vi "PhDemoLV.vi"() -> ()   [LabVIEW 2013]
doc: "This is an example VI that demonstrates a few capabilities of the Vision Research Phantom Series LabVIEW Driver."
uses:
  _Type Defs/enum buttons.ctl
  _Type Defs/Point.ctl
  _Type Defs/StampTime.ctl
  _Type Defs/Cine Source.ctl
  _Type Defs/PHCon ACQUIPARAMS.ctl
  _Type Defs/PhCon SyncImaging.ctl
  _Type Defs/Rect.ctl
  _Type Defs/PHCon Time64.ctl
  _Type Defs/PhInt CFA.ctl
  _Type Defs/PhCon Predefined Cines.ctl
  _Type Defs/PhFile InfName.ctl
  _Type Defs/PHCon IMRANGE.ctl
  _Type Defs/PhInt PhProcessImage Selectors.ctl
  Instance          21 27Saved   Application Example .vi
  VRI.lvlib
panel:
  out "Parameters":T1 {"CFA"."CFA" items=["CFA_NONE", "CFA_VRI", "CFA_VRIV6", "CFA_BAYER", "CFA_BAYERFLIP"]; "TriggerTime"."fractions" format="%32.0f"}
  in  "Cine Number":i32=1 max=1
  out "Current Image #":i32
  out "Slide":dbl(slide) scale=0.0..1.0
  in  "Play/Pause":bool
  in  "Preview Img":bool
  in  "Delay (ms)":u32=10
  out "Image Count":u32
  out "Post-Trigger Frames":i32
  in  "Source":T6 items=["Camera RAM", "File"]
  in  "Save Cine":bool
  in  "Open Cine":bool
  in  "Trigger":bool
  in  "Capture":bool
  in  "EXIT":bool
  out "pCameraName":string
  out "pSerial":u32
  in  "Update":bool
  in  "ACQUIPARAMS Display":T7
  in  "Save StampTime":T8
  out "Preview":picture
  out "Continue":bool
  out "Save Progress":u8(slide) max=100 scale=0.0..100.0
  out "active":string="Not Running..."
  out "CAR":T9[](array[typedef])
  in  "Camera Number":u32
  out "error out":errorcluster
  in  "error in":errorcluster
  in  "Current State":T10
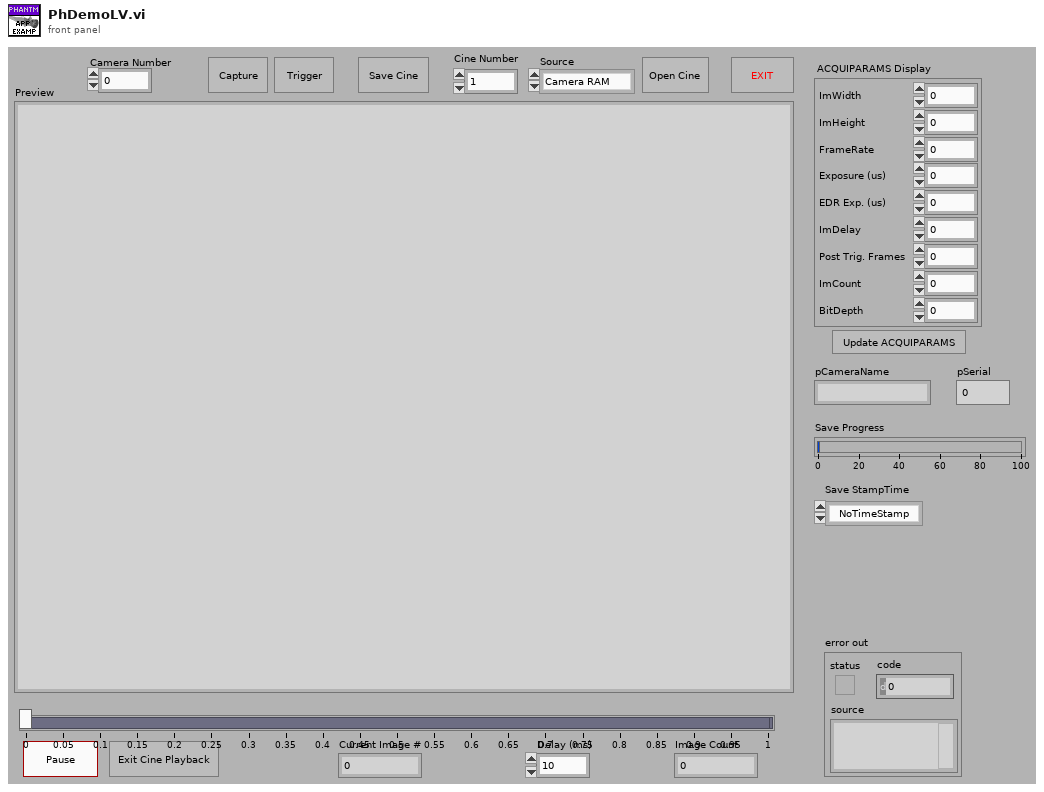
[diagram p1: front panel]
types:
  T1 = typedef "VRI.lvlib/PHCon ACQUIPARAMS.ctl" = cluster{"ImWidth":u32, "ImHeight":u32, "(deprecated)FrameRateInt":u32, "Exposure":u32, "EDRExposure":u32, "ImDelay":u32, "PTFrames":u32, "ImCount":u32, "SyncImaging":T2, "AutoExposure":u32, "AutoExpLevel":u32, "AutoExpSpeed":u32, "AutoExpRect":T3, "Recorded":bool, "TriggerTime":T4, "RecordedCount":u32, "FirstIm":i32, "FRPSteps":u32, "FRPImgNr":i32[], "FRPRate":u32[], "FRPExp":u32[], "Decimation":u32, "BitDepth":u32, "CamGainRed":u32, "CamGainGreen":u32, "CamGainBlue":u32, "CamGain":u32, "ShutterOff":bool, "CFA":T5, "CineName[256]":u8[], "Description[4096]":u8[], "FRPShape [16]":u32[], "dFrameRate":dbl}
  T2 = typedef "VRI.lvlib/PhCon SyncImaging.ctl" = enum32{"SYNC_INTERNAL", "SYNC_EXTERNAL", "SYNC_LOCKTOIRIG"}
  T3 = typedef "VRI.lvlib/Rect.ctl" = cluster{"X":i32, "Y":i32, "Width":i32, "Height":i32}
  T4 = typedef "VRI.lvlib/PHCon Time64.ctl" = cluster{"fractions":u32, "seconds":u32}
  T5 = typedef "VRI.lvlib/PhInt CFA.ctl" = cluster{"CFA":u32, "VRIV6 Mask":cluster{"TL_GRAY":bool, "TR_GRAY":bool, "BL_GRAY":bool, "BR_GRAY":bool}}
  T6 = typedef "VRI.lvlib/Cine Source.ctl" = u16
  T7 = cluster{"ImWidth":u32, "ImHeight":u32, "FrameRate":u32, "Exposure (us)":u32, "EDR Exp. (us)":u32, "ImDelay":u32, "Post Trig. Frames":u32, "ImCount":u32, "BitDepth":u32}
  T8 = typedef "VRI.lvlib/StampTime.ctl" = enum32{"NoTimeStamp", "Time stamp", "", "Time stamp from trigger"}
  T9 = typedef "VRI.lvlib/Point.ctl" = cluster{"X":i32, "Y":i32}
  T10 = typedef "VRI.lvlib/enum buttons.ctl" = enum16{"Initialize", "Wait for Action", "Update", "Capture", "Trigger", "Open Cine", "Save Cine", "End"}
  T11 = typedef "VRI.lvlib/PHCon IMRANGE.ctl" = cluster{"First":i32, "Cnt":u32}
  T12 = typedef "VRI.lvlib/PhCon Predefined Cines.ctl" = i32
  T13 = typedef "VRI.lvlib/PhInt PhProcessImage Selectors.ctl" = u16
  T14 = typedef "VRI.lvlib/PhFile InfName.ctl" = u32
  T15 = typedef "VRI.lvlib/PhInt IH.ctl" = cluster{"biSize":u32, "biWidth":i32, "biHeight":i32, "biPlanes":u16, "biBitCount":u16, "biCompresssion":u32, "biSizeImage":u32, "biXPelsPerMeter":i32, "biYPelsPerMeter":i32, "biClrUsed":u32, "biClrImportant":u32, "BlackLevel":i32, "WhiteLevel":i32}
  T16 = typedef "VRI.lvlib/BITMAPINFOHEADER.ctl" = cluster{"biSize":u32, "biWidth":i32, "biHeight":i32, "biPlanes":u16, "biBitCount":u16, "biCompression":u32, "biSizeImage":u32, "biXPelsPerMeter":i32, "biYPelsPerMeter":i32, "biClrUsed":u32, "biClrImportant":u32}
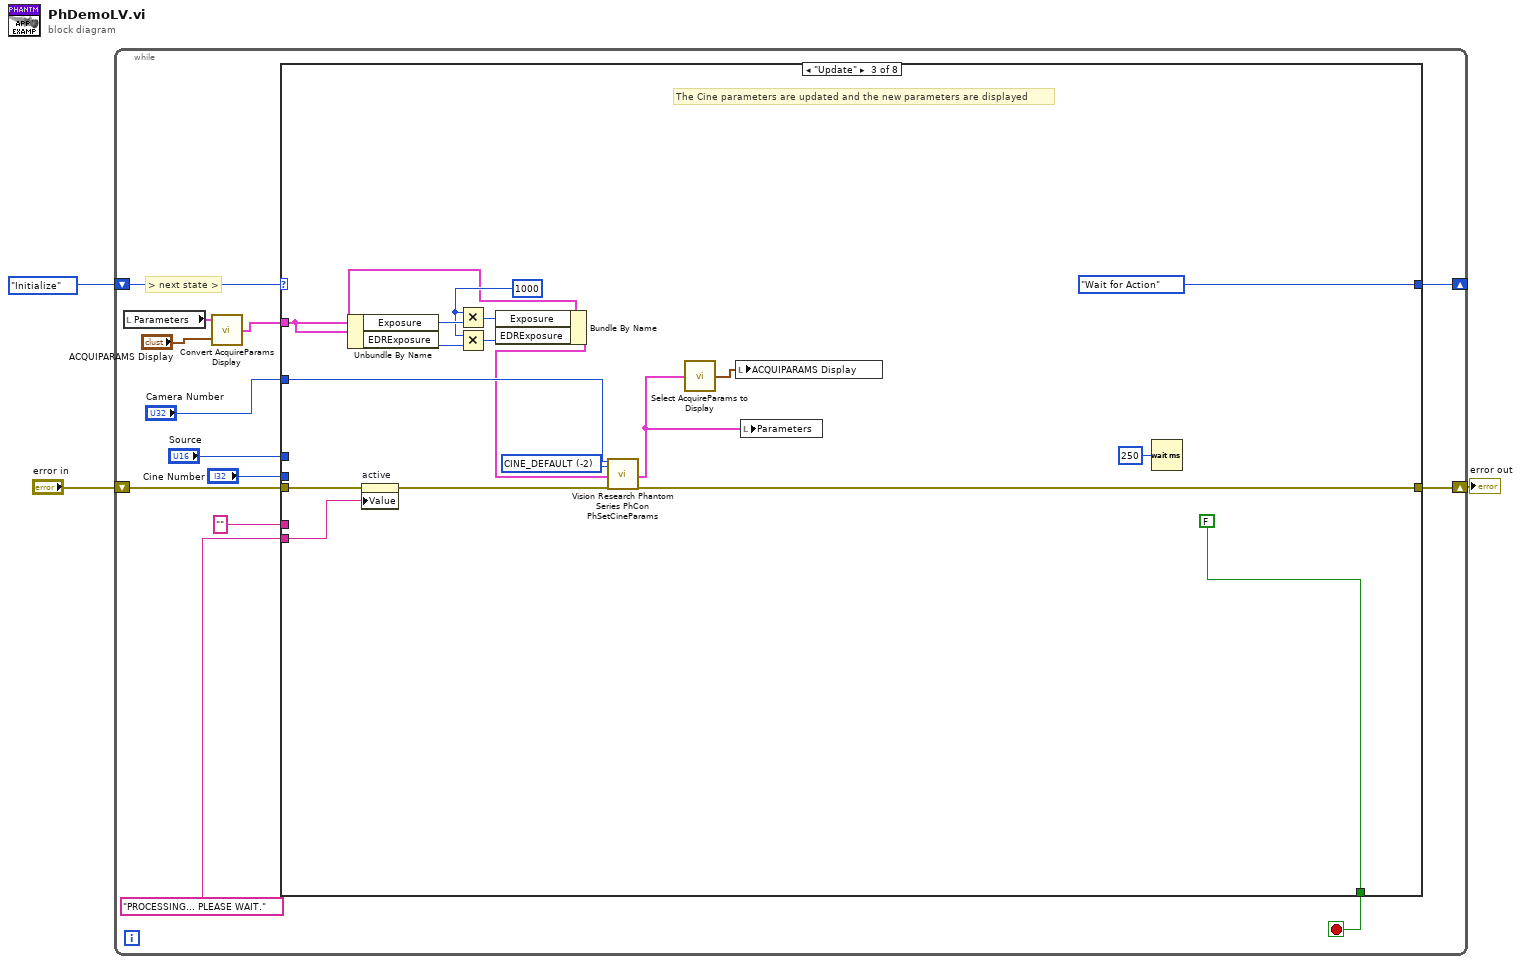
[diagram p0: block diagram]
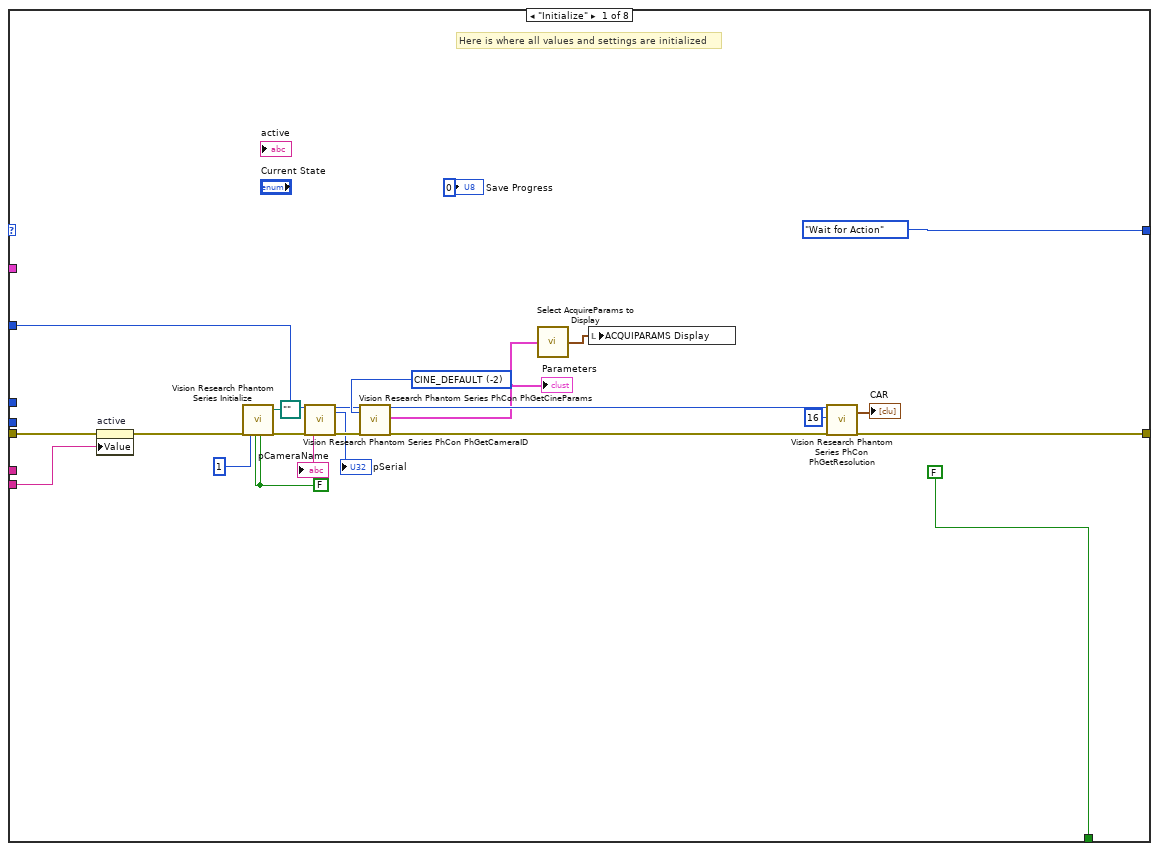
[diagram p2: hidden frame]
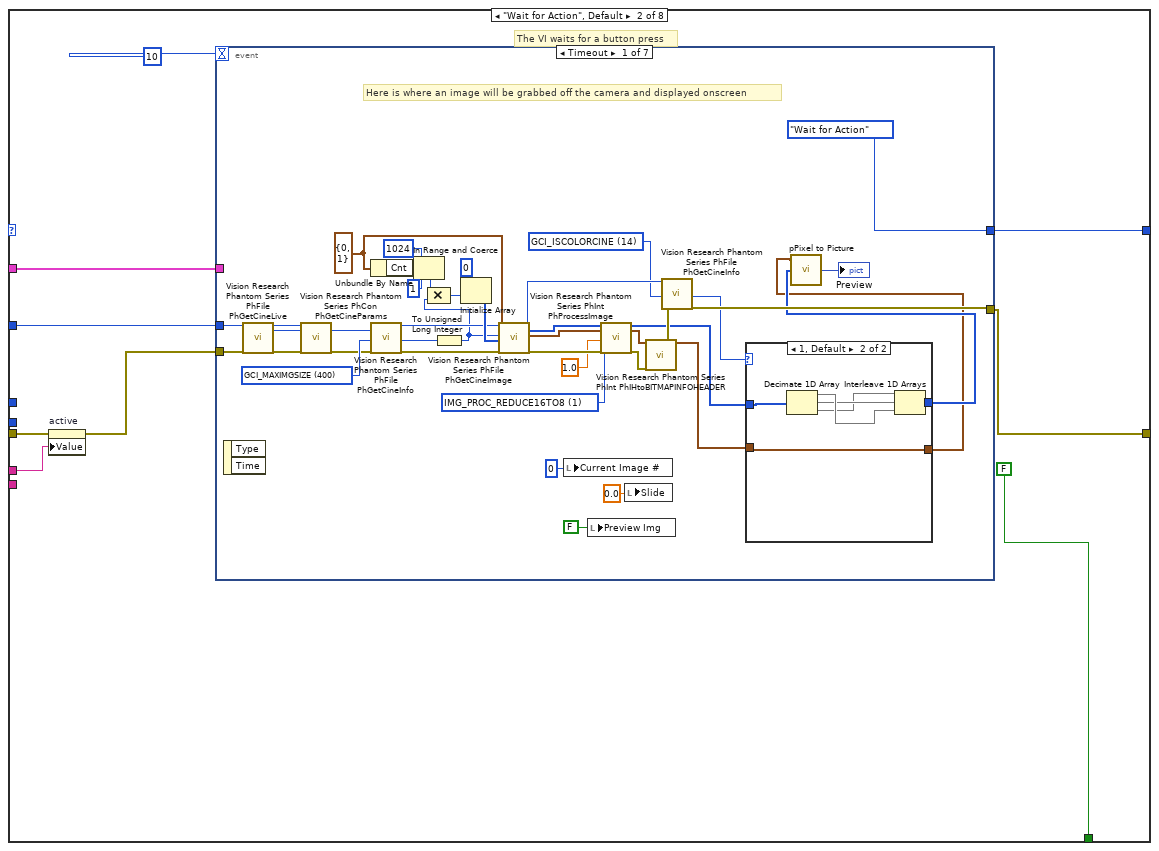
[diagram p3: hidden frame]
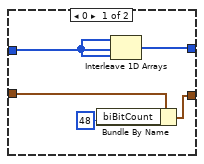
[diagram p4: hidden frame]
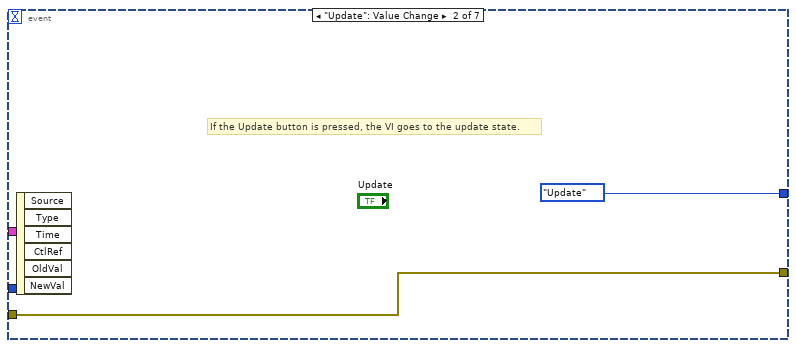
[diagram p5: hidden frame]
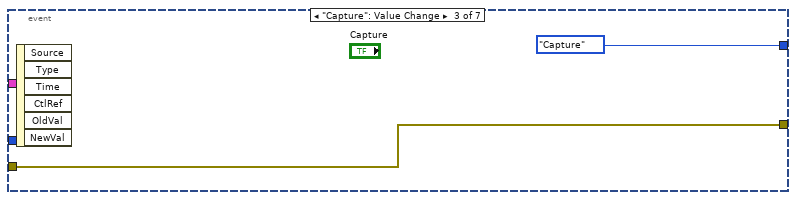
[diagram p6: hidden frame]
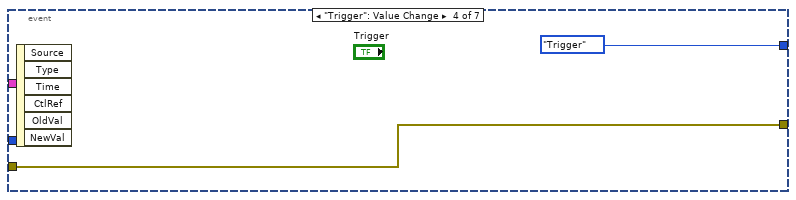
[diagram p7: hidden frame]
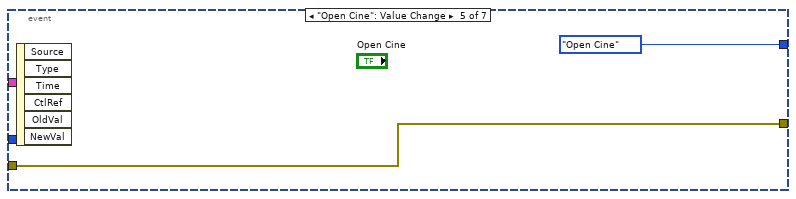
[diagram p8: hidden frame]
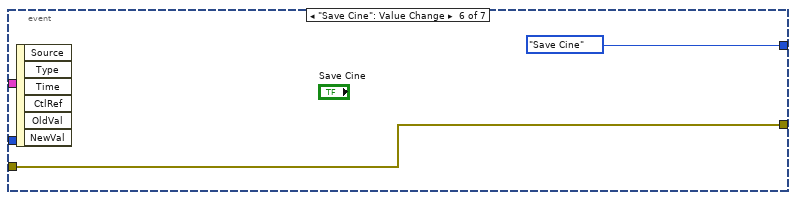
[diagram p9: hidden frame]
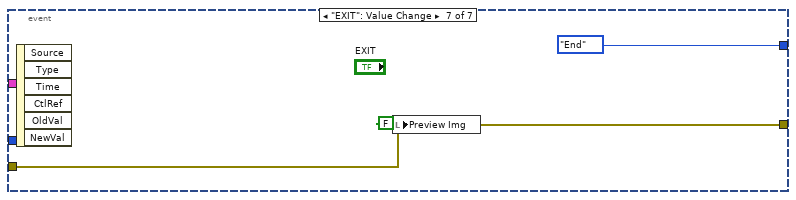
[diagram p10: hidden frame]
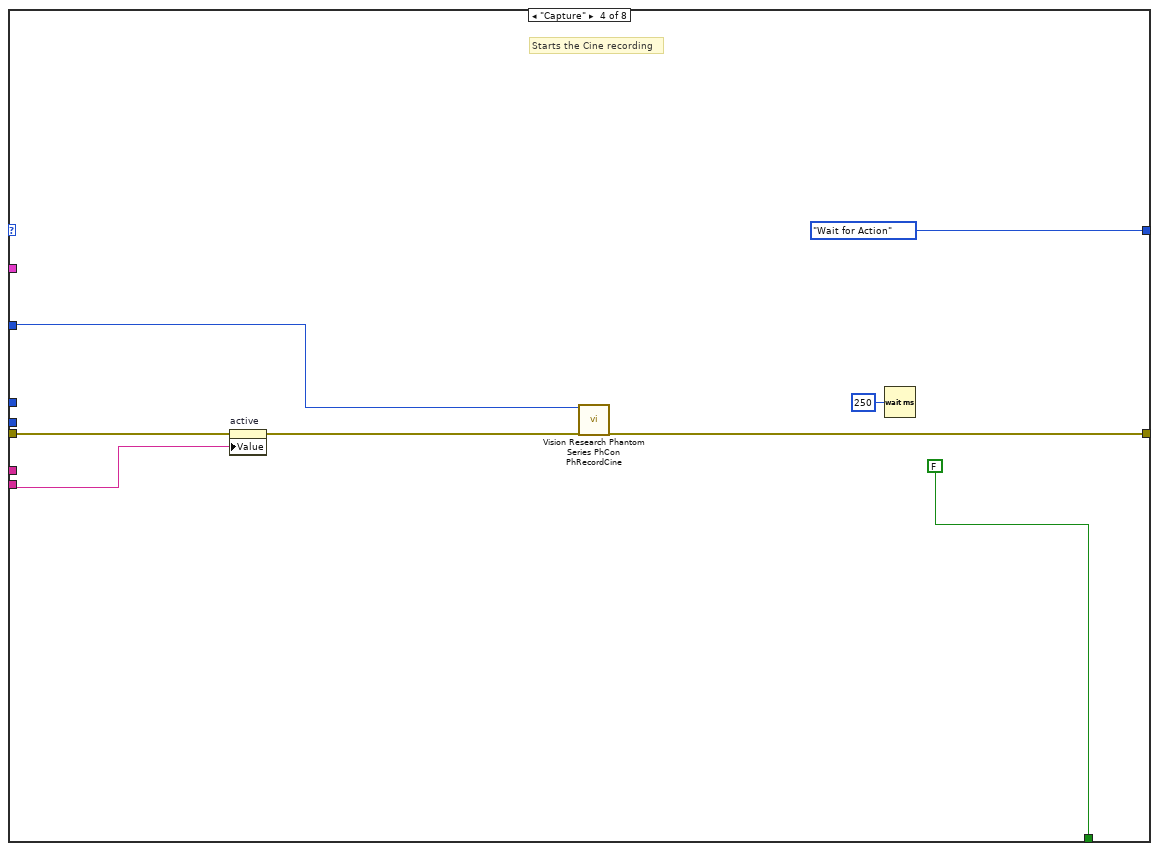
[diagram p11: hidden frame]
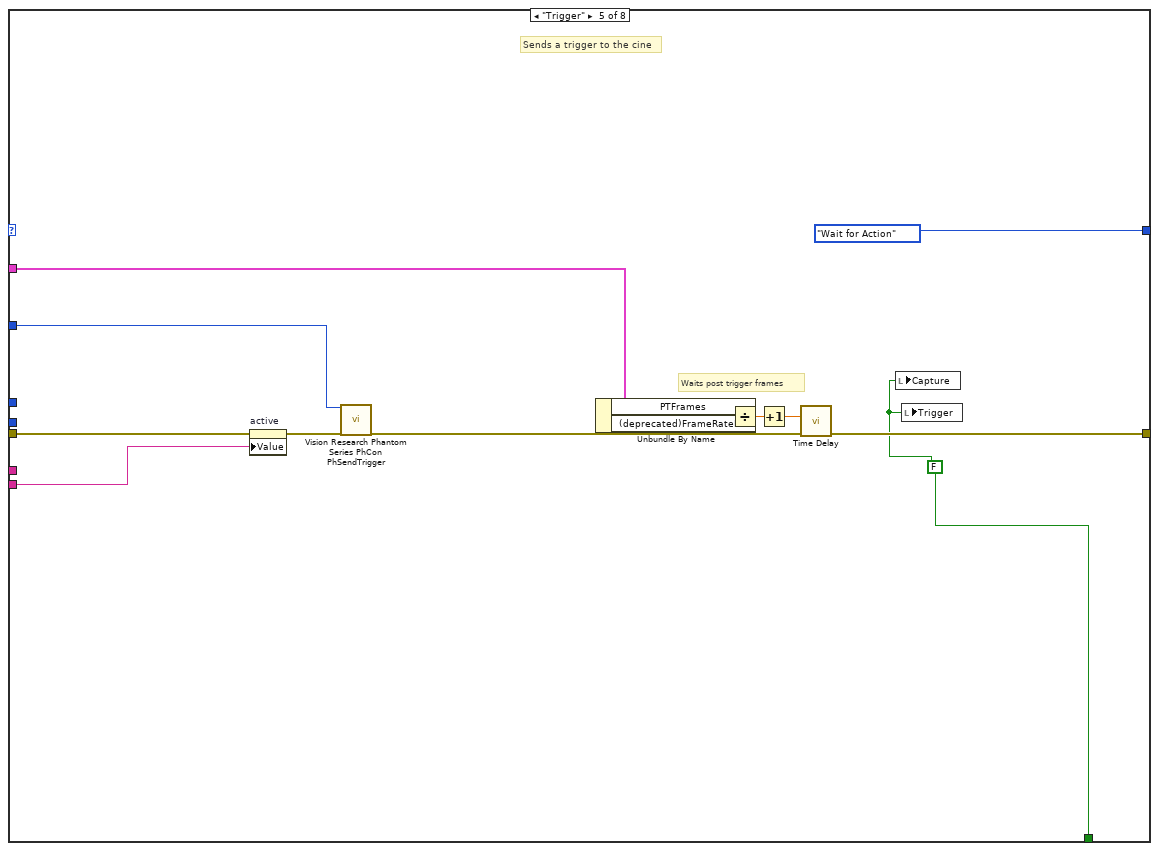
[diagram p12: hidden frame]
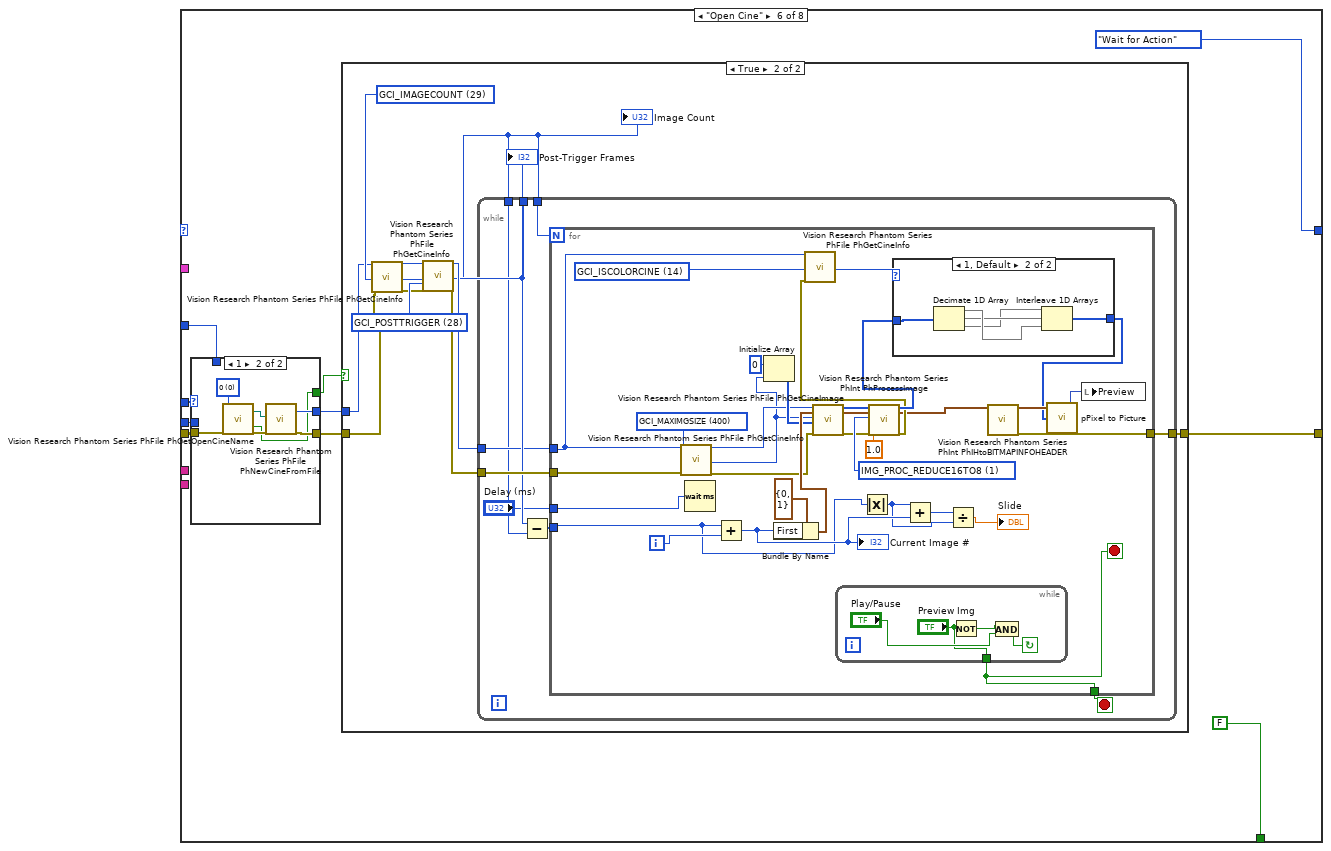
[diagram p13: hidden frame]
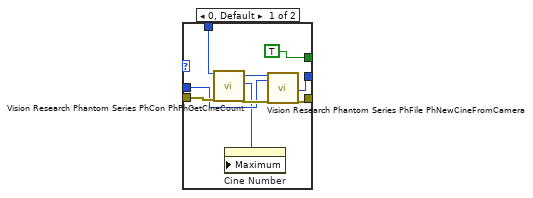
[diagram p16: hidden frame]
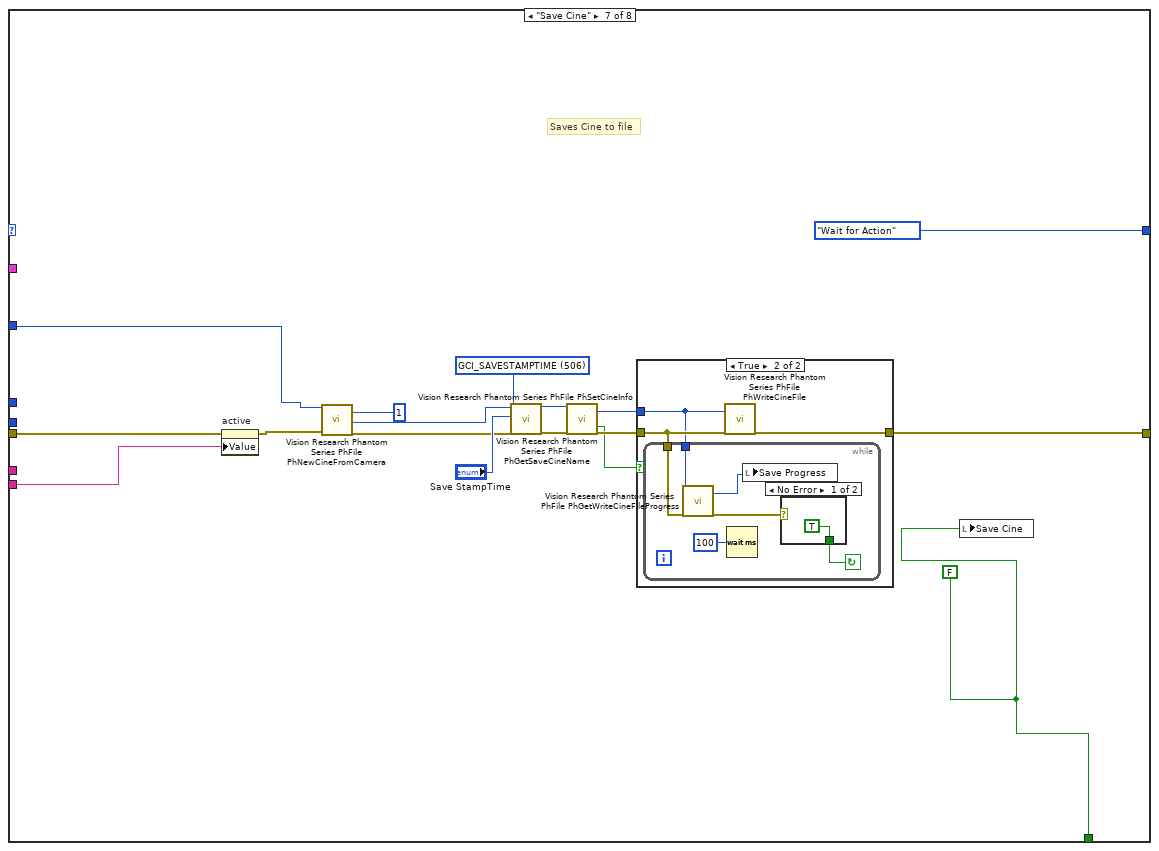
[diagram p17: hidden frame]
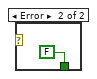
[diagram p19: hidden frame]
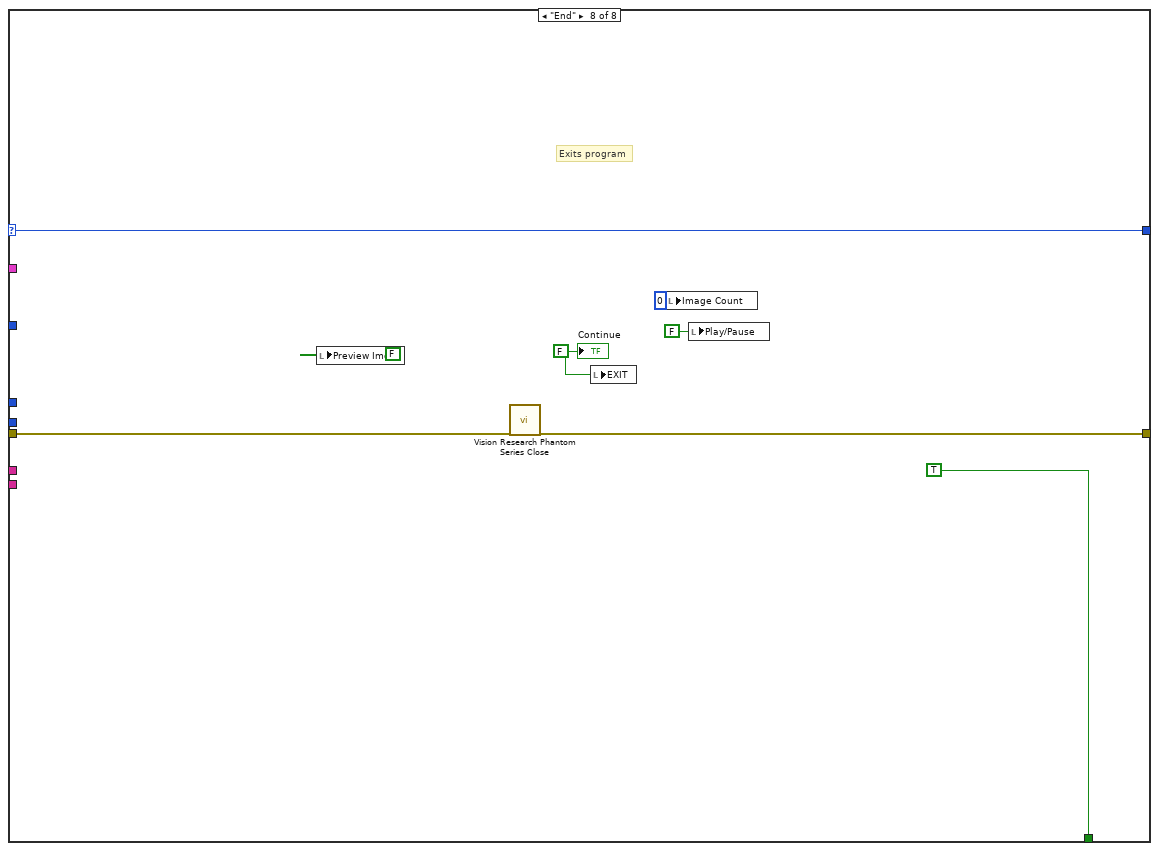
[diagram p20: hidden frame]
diagram:
  n1 = while {
    shift-right: [w16] -> _
    shift-left: enum_buttons."Initialize" ("Enum") -> [w15]
    shift-right: [w13] -> w2
    shift-left: "error in" -> [w10]
    stop <- w14 stop-if-true
    # "> next state >"
    n2 = local read "Parameters"() -> (w4:T1)
    n3 = call "Convert AcquireParams Display.vi"("ACQUIPARAMS Display"="ACQUIPARAMS Display", "ACQUIPARAMS [in]"=w4) -> ("ACQUIPARAMS [out]"=w8:T1)
    n4 = case shown="\"Update\"" w15 {
      selector: w15 -> [_ _ _ _ _ _ _ w277]
      tunnel: w8 -> [_ w44 w117 _ w145 _ _ _]
      tunnel: [enum_buttons."Wait for Action" ("Enum") w47 enum_buttons."Wait for Action" ("Enum") enum_buttons."Wait for Action" ("Enum") enum_buttons."Wait for Action" ("Enum") enum_buttons."Wait for Action" ("Enum") enum_buttons."Wait for Action" ("Enum") w277] -> w16
      tunnel: [FALSE FALSE FALSE FALSE w139 FALSE w241 TRUE] -> w14
      tunnel: w10 -> [w26 w42 w127 w135 w150 w159 w256 w275]
      tunnel: [w38 w45 w115 w137 w142 w156 w245 w274] -> w13
      tunnel: "PROCESSING... PLEASE WAIT." ("active") -> [w24 _ w125 w134 w148 _ w255 _]
      tunnel: "" ("active") -> [_ w43 _ _ _ _ _ _]
      tunnel: "Camera Number" -> [w22 w41 w123 w131 w140 w154 w247 _]
      tunnel: "Source" -> [_ _ _ _ _ w155 _ _]
      tunnel: "Cine Number" -> [_ _ _ _ _ w153 _ _]
      frame "Initialize" {
        w30 = FALSE ("ID Query (T: Check)")
        w33 = T12 -2 items=["CINE_DEFAULT "=-2, "CINE_CURRENT "=-1, "CINE_PREVIEW  "=0, "CINE_FIRST    "=1] ("Cine")
        # "Here is where all values and settings are initialized"
        n5 = property on="active" class="Str"(error in=w26, "Value"=w24) -> (error out=w25:errorcluster)  [unwired: 1 in, 1 out]
        n6 = call "Vision Research Phantom Series Initialize.vi"("Storage Path (\"\")"=path "" ("Storage Path (\"\")"), "error in (no error)"=w25, "CallID"=u32 1, "ID Query (T: Check)"=w30, "Reset (F: Don't Reset)"=w30) -> ("Error Out"=w29:errorcluster)  [unwired: 14 out]
        n7 = call "Vision Research Phantom Series PhCon PhGetCameraID.vi"("CN in"=w22, "Error In (no error)"=w29) -> ("CN out"=w28:u32, "pSerial"=→"pSerial":u32, "pCameraName"=→"pCameraName":string, "Error Out"=w27:errorcluster)  [unwired: 14 out]
        n8 = call "Vision Research Phantom Series PhCon PhGetCineParams.vi"("CN in"=w28, "Cine"=w33, "Error In (no error)"=w27) -> ("CN out"=w36:u32, "ACQUIPARAMS"=w20:T1, "Error Out"=w21:errorcluster)  [unwired: 14 out]
        "Parameters" <- w20
        n9 = call "Select AcquireParams to Display.vi"("ACQUIPARAMS"=w20) -> ("ACQUIPARAMS Display"=w19:T7)
        n10 = local write "ACQUIPARAMS Display"(w19) -> ()
        n11 = call "Vision Research Phantom Series PhCon PhGetResolution.vi"("CN in"=w36, "pCnt"=16, "Error In (no error)"=w21) -> ("CAR"=→"CAR":T9[], "Error Out"=w38:errorcluster)  [unwired: 1 in, 14 out]
        "Save Progress" <- u8 0 ("Value")
      }
      frame "Wait for Action", Default {
        # "The VI waits for a button press"
        n12 = property on="active" class="Str"(error in=w42, "Value"=w43) -> (error out=w40:errorcluster)  [unwired: 1 in, 1 out]
        n13 = event shown="[0] Timeout" {
          selector: _ -> [_ _ _ _ _ _ _]
          dyn-events: _ -> [_ _ _ _ _ _ _]
          timeout: 10 -> [_ _ _ _ _ _ _]
          tunnel: [enum_buttons."Wait for Action" ("Enum") enum_buttons."Update" ("Enum") enum_buttons."Capture" ("Enum") enum_buttons."Trigger" ("Enum") enum_buttons."Open Cine" ("Enum") enum_buttons."Save Cine" ("Enum") enum_buttons."End" ("Enum")] -> w47
          tunnel: w40 -> [w68 w100 w102 w104 w107 w108 w111]
          tunnel: [w55 w100 w102 w104 w107 w108 w111] -> w45
          tunnel: w44 -> [_ _ _ _ _ _ _]
          tunnel: w41 -> [w64 _ _ _ _ _ _]
          event Timeout {
            w60 = T13 1 items=["IMG_PROC_REDUCE16TO8"=1] ("procID")
            w86 = T11 {"First"=0, "Cnt"=1} ("pRng")
            w62 = T14 14 items=["GCI_CFA"=0, "GCI_FRAMERATE"=1, "GCI_EXPOSURE"=2, "GCI_AUTOEXPOSURE"=3, "GCI_REALBPP"=4, "GCI_CAMERASERIAL"=5, "GCI_HEADSERIAL0"=6, "GCI_HEADSERIAL1"=7, "GCI_HEADSERIAL2"=8, "GCI_HEADSERIAL3"=9, "GCI_TRIGTIMESEC"=10, "GCI_TRIGTIMEFR"=11, "GCI_ISFILECINE"=12, "GCI_IS16BPPCINE"=13, "GCI_ISCOLORCINE"=14, "GCI_ISMULTIHEADCINE"=15, "GCI_EXPOSURENS"=16, "GCI_EDREXPOSURENS"=17, "GCI_FRAMEDELAYNS"=19, "GCI_FROMFILETYPE"=20, "GCI_COMPRESSION"=21, "GCI_CAMERAVERSION"=22, "GCI_ROTATE"=23, "GCI_IMWIDTH"=24, "GCI_IMHEIGHT"=25, "GCI_IMWIDTHACQ"=26, "GCI_IMHEIGHTACQ"=27, "GCI_POSTTRIGGER"=28, "GCI_IMAGECOUNT"=29, "GCI_TOTALIMAGECOUNT"=30, "GCI_TRIGFRAME"=31, "GCI_AUTOEXPLEVEL"=32, "GCI_AUTOEXPTOP"=33, "GCI_AUTOEXPLEFT"=34, "GCI_AUTOEXPBOTTOM"=35, "GCI_AUTOEXPRIGHT"=36, "GCI_RECORDINGTIMEZONE"=37, "GCI_FIRSTIMAGENO"=38, "GCI_FIRSTMOVIEIMAGE"=39, "GCI_CINENAME"=40, "GCI_FRPSTEPS"=100, "GCI_FRP1X"=101, "GCI_FRP1Y"=102, "GCI_FRP2X"=103, "GCI_FRP2Y"=104, "GCI_FRP3X"=105, "GCI_FRP3Y"=106, "GCI_FRP4X"=107, "GCI_FRP4Y"=108, "GCI_WRITEERR"=109, "GCI_LENSDESCRIPTION"=110, "GCI_LENSAPERATURE"=111, "GCI_LENSFOCALLENGTH"=112, "GCI_WB"=200, "GCI_WBVIEW"=201, "GCI_BRIGHT"=202, "GCI_CONTRAST"=203, "GCI_GAMMA"=204, "GCI_GAMMAR"=223, "GCI_GAMMAB"=224, "GCI_SATURATION"=205, "GCI_HUE"=206, "GCI_FLIPH"=207, "GCI_FLIPV"=208, "GCI_FILTERCODE"=209, "GCI_IMFILTER"=210, "GCI_INTALGO"=211, "GCI_PEDESTALR"=212, "GCI_PEDESTALG"=213, "GCI_PEDESTALB"=214, "GCI_FLARE"=225, "GCI_CHROMA"=226, "GCI_TONE"=227, "GCI_ENABLEMATRICES"=228, "GCI_USERMATRIX"=229, "GCI_RESAMPLEACTIVE"=215, "GCI_RESAMPLEWIDTH"=216, "GCI_RESAMPLEHEIGHT"=217, "GCI_CROPACTIVE"=218, "GCI_CROPRECTANGLE"=219, "GCI_OFFSET16_8"=220, "GCI_GAIN16_8"=221, "GCI_DEMOSAICINGFUNCPTR"=222, "GCI_VFLIPVIEWACTIVE"=300, "GCI_MAXIMGSIZE"=400, "GCI_FRPIMGNOARRAY"=450, "GCI_FRPRATEARRAY"=451, "GCI_FRPSHAPEARRAY"=452, "GCI_TRIGTC"=470, "GCI_TRIGTCU"=471, "GCI_PBRATE"=472, "GCI_TCRATE"=473, "GCI_SAVERANGE"=500, "GCI_SAVEFILENAME"=501, "GCI_SAVEFILETYPE"=502, "GCI_SAVE16BIT"=503, "GCI_SAVEPACKED"=504, "GCI_SAVEXML"=505, "GCI_SAVESTAMPTIME"=506, "GCI_SAVEAVIFRAMERATE"=520, "GCI_SAVEAVICOMPRESSORLIST"=521, "GCI_SAVEAVICOMPRESSORINDEX"=522, "GCI_SAVEDPXLSB"=530, "GCI_SAVEDPXTO10BPS"=531, "GCI_SAVEDPXDATAPACKING"=532, "GCI_SAVEDPX10BITLOG"=533, "GCI_SAVEDPXEXPORTLOGLUT"=534, "GCI_SAVEDPX10BITLOGREFWHITE"=535, "GCI_SAVEDPX10BITLOGREFBLACK"=536, "GCI_SAVEDPX10BITLOGGAMMA"=537, "GCI_SAVEDPX10BITLOGFILMGAMMA"=538, "GCI_SAVEQTPLAYBACKRATE"=550, "GCI_SAVECCIQUALITY"=560, "GCI_UNCALIBRATEDIMAGE"=600, "GCI_NOPROCESSING"=601, "GCI_BADPIXELREPAIR"=602] ("InfName")
            w87 = T14 400 items=["GCI_CFA"=0, "GCI_FRAMERATE"=1, "GCI_EXPOSURE"=2, "GCI_AUTOEXPOSURE"=3, "GCI_REALBPP"=4, "GCI_CAMERASERIAL"=5, "GCI_HEADSERIAL0"=6, "GCI_HEADSERIAL1"=7, "GCI_HEADSERIAL2"=8, "GCI_HEADSERIAL3"=9, "GCI_TRIGTIMESEC"=10, "GCI_TRIGTIMEFR"=11, "GCI_ISFILECINE"=12, "GCI_IS16BPPCINE"=13, "GCI_ISCOLORCINE"=14, "GCI_ISMULTIHEADCINE"=15, "GCI_EXPOSURENS"=16, "GCI_EDREXPOSURENS"=17, "GCI_FRAMEDELAYNS"=19, "GCI_FROMFILETYPE"=20, "GCI_COMPRESSION"=21, "GCI_CAMERAVERSION"=22, "GCI_ROTATE"=23, "GCI_IMWIDTH"=24, "GCI_IMHEIGHT"=25, "GCI_IMWIDTHACQ"=26, "GCI_IMHEIGHTACQ"=27, "GCI_POSTTRIGGER"=28, "GCI_IMAGECOUNT"=29, "GCI_TOTALIMAGECOUNT"=30, "GCI_TRIGFRAME"=31, "GCI_AUTOEXPLEVEL"=32, "GCI_AUTOEXPTOP"=33, "GCI_AUTOEXPLEFT"=34, "GCI_AUTOEXPBOTTOM"=35, "GCI_AUTOEXPRIGHT"=36, "GCI_RECORDINGTIMEZONE"=37, "GCI_FIRSTIMAGENO"=38, "GCI_FIRSTMOVIEIMAGE"=39, "GCI_CINENAME"=40, "GCI_FRPSTEPS"=100, "GCI_FRP1X"=101, "GCI_FRP1Y"=102, "GCI_FRP2X"=103, "GCI_FRP2Y"=104, "GCI_FRP3X"=105, "GCI_FRP3Y"=106, "GCI_FRP4X"=107, "GCI_FRP4Y"=108, "GCI_WRITEERR"=109, "GCI_LENSDESCRIPTION"=110, "GCI_LENSAPERATURE"=111, "GCI_LENSFOCALLENGTH"=112, "GCI_WB"=200, "GCI_WBVIEW"=201, "GCI_BRIGHT"=202, "GCI_CONTRAST"=203, "GCI_GAMMA"=204, "GCI_GAMMAR"=223, "GCI_GAMMAB"=224, "GCI_SATURATION"=205, "GCI_HUE"=206, "GCI_FLIPH"=207, "GCI_FLIPV"=208, "GCI_FILTERCODE"=209, "GCI_IMFILTER"=210, "GCI_INTALGO"=211, "GCI_PEDESTALR"=212, "GCI_PEDESTALG"=213, "GCI_PEDESTALB"=214, "GCI_FLARE"=225, "GCI_CHROMA"=226, "GCI_TONE"=227, "GCI_ENABLEMATRICES"=228, "GCI_USERMATRIX"=229, "GCI_RESAMPLEACTIVE"=215, "GCI_RESAMPLEWIDTH"=216, "GCI_RESAMPLEHEIGHT"=217, "GCI_CROPACTIVE"=218, "GCI_CROPRECTANGLE"=219, "GCI_OFFSET16_8"=220, "GCI_GAIN16_8"=221, "GCI_DEMOSAICINGFUNCPTR"=222, "GCI_VFLIPVIEWACTIVE"=300, "GCI_MAXIMGSIZE"=400, "GCI_FRPIMGNOARRAY"=450, "GCI_FRPRATEARRAY"=451, "GCI_FRPSHAPEARRAY"=452, "GCI_TRIGTC"=470, "GCI_TRIGTCU"=471, "GCI_PBRATE"=472, "GCI_TCRATE"=473, "GCI_SAVERANGE"=500, "GCI_SAVEFILENAME"=501, "GCI_SAVEFILETYPE"=502, "GCI_SAVE16BIT"=503, "GCI_SAVEPACKED"=504, "GCI_SAVEXML"=505, "GCI_SAVESTAMPTIME"=506, "GCI_SAVEAVIFRAMERATE"=520, "GCI_SAVEAVICOMPRESSORLIST"=521, "GCI_SAVEAVICOMPRESSORINDEX"=522, "GCI_SAVEDPXLSB"=530, "GCI_SAVEDPXTO10BPS"=531, "GCI_SAVEDPXDATAPACKING"=532, "GCI_SAVEDPX10BITLOG"=533, "GCI_SAVEDPXEXPORTLOGLUT"=534, "GCI_SAVEDPX10BITLOGREFWHITE"=535, "GCI_SAVEDPX10BITLOGREFBLACK"=536, "GCI_SAVEDPX10BITLOGGAMMA"=537, "GCI_SAVEDPX10BITLOGFILMGAMMA"=538, "GCI_SAVEQTPLAYBACKRATE"=550, "GCI_SAVECCIQUALITY"=560, "GCI_UNCALIBRATEDIMAGE"=600, "GCI_NOPROCESSING"=601, "GCI_BADPIXELREPAIR"=602] ("InfName")
            # "Here is where an image will be grabbed off the camera and displayed onscreen"
            n14 = event-data() -> ()  [unwired: 3 out]
            n15 = call "Vision Research Phantom Series PhFile PhGetCineLive.vi"("CN (in)"=w64, "Error In (no error)"=w68) -> ("CN (out)"=w80:u32, "pCH (out)"=w70:u32, "Error Out"=w78:errorcluster)  [unwired: 15 out]
            n16 = call "Vision Research Phantom Series PhCon PhGetCineParams.vi"("CN in"=w80, "Error In (no error)"=w78) -> ("Error Out"=w79:errorcluster)  [unwired: 1 in, 16 out]
            n17 = Unbundle By Name(w86) -> ("Cnt"=w81:u32)
            n18 = call "Vision Research Phantom Series PhFile PhGetCineInfo.vi"("CH in"=w70, "InfName"=w87, "Error In (no error)"=w79) -> ("CH out"=w72:u32, "pInfVal out"=w71:i32, "Error Out"=w74:errorcluster)  [unwired: 14 out]
            n19 = In Range and Coerce(upper limit=u32 1024, x=w81, lower limit=u32 1) -> (coerced(x)=w82:u32)  [unwired: 1 out]
            n20 = To Unsigned Long Integer(number=w71) -> (unsigned 32bit integer=w54:u32)
            n21 = Compound Arithmetic op=MULTIPLY(w82, w54) -> (w85:u32)
            n22 = Initialize Array(u16 0 ("element"), w85) -> (w73:u16[])
            n23 = call "Vision Research Phantom Series PhFile PhGetCineImage.vi"("hC [in]"=w72, "pRng [in]"=w86, "bufferByteSize [in]"=w54, "pPixelBuffer [in]"=w73, "Error In (no error)"=w74) -> ("hC [out]"=w63:u32, "pPixelBuffer [out]"=w75:u16[], "IH [out]"=w76:T15, "Error Out"=w77:errorcluster)  [unwired: 11 out]
            n24 = local write "Current Image #"(0 ("Current Image #")) -> ()
            n25 = local write "Preview Img"(FALSE ("Preview Img")) -> ()
            n26 = call "Vision Research Phantom Series PhInt PhProcessImage.vi"("pPixelSrc [in]"=w75, "IH [in]"=w76, "procID"=w60, "pProcParams"=1.0, "Error In (no error)"=w77) -> ("pPixelDest [out]"=w52:u8[], "IH [out]"=w66:T15, "Error Out"=w65:errorcluster)  [unwired: 12 out]
            n27 = local write "Slide"(0.0 ("Slide")) -> ()
            n28 = call "Vision Research Phantom Series PhInt PhIHtoBITMAPINFOHEADER.vi"("IH"=w66, "Error In (no error)"=w65) -> ("BITMAPINFOHEADER"=w50:T16, "Error Out"=w56:errorcluster)  [unwired: 16 out]
            n29 = call "Vision Research Phantom Series PhFile PhGetCineInfo.vi"("CH in"=w63, "InfName"=w62, "Error In (no error)"=w56) -> ("pInfVal out"=w53:i32, "Error Out"=w55:errorcluster)  [unwired: 15 out]
            n30 = case shown="1, Default" w53 {
              tunnel: [w91 w96] -> w51
              tunnel: w52 -> [w92 w95]
              tunnel: w50 -> [w90 w94]
              tunnel: [w89 w94] -> w49
              frame 0 {
                n31 = Bundle By Name(cluster=w90, "biBitCount"=u16 48) -> (w89:T16)
                n32 = Interleave 1D Arrays(w92, w92, w92) -> (w91:u8[])
              }
              frame 1, Default {
                n33 = Decimate 1D Array(w95) -> (w99:u8[], w98:u8[], w97:u8[])
                n34 = Interleave 1D Arrays(w97, w98, w99) -> (w96:u8[])
              }
            }
            n35 = call "pPixel to Picture.vi"("pPixel"=w51, "BITMAPINFOHEADER"=w49) -> ("Preview"=→"Preview":picture)  [unwired: 1 in]
          }
          event "Update": Value Change {
            # "If the Update button is pressed, the VI goes to the update state."
            n36 = event-data() -> ()  [unwired: 7 out]
          }
          event "Capture": Value Change {
            n37 = event-data() -> ()  [unwired: 7 out]
          }
          event "Trigger": Value Change {
            n38 = event-data() -> ()  [unwired: 7 out]
          }
          event "Open Cine": Value Change {
            n39 = event-data() -> ()  [unwired: 7 out]
          }
          event "Save Cine": Value Change {
            n40 = event-data() -> ()  [unwired: 7 out]
          }
          event "EXIT": Value Change {
            n41 = event-data() -> ()  [unwired: 7 out]
            n42 = local write "Preview Img"(FALSE ("Preview Img")) -> ()
          }
        }
      }
      frame "Update" {
        w120 = u32 1000 ("x")
        w128 = T12 -2 items=["CINE_DEFAULT "=-2, "CINE_CURRENT "=-1, "CINE_PREVIEW  "=0, "CINE_FIRST    "=1] ("Cine")
        # "The Cine parameters are updated and the new parameters are displayed"
        n43 = Unbundle By Name(w117) -> ("Exposure"=w122:u32, "EDRExposure"=w121:u32)
        n44 = property on="active" class="Str"(error in=w127, "Value"=w125) -> (error out=w126:errorcluster)  [unwired: 1 in, 1 out]
        n45 = Multiply(x=w120, y=w122) -> (x*y=w119:u32)
        n46 = Multiply(x=w120, y=w121) -> (x*y=w118:u32)
        n47 = Bundle By Name(cluster=w117, "Exposure"=w119, "EDRExposure"=w118) -> (w116:T1)
        n48 = call "Vision Research Phantom Series PhCon PhSetCineParams.vi"("CN in"=w123, "Cine"=w128, "ACQUIPARAMS"=w116, "Error In (no error)"=w126) -> ("ACQUIPARAMS out"=w113:T1, "Error Out"=w115:errorcluster)  [unwired: 14 out]
        n49 = call "Select AcquireParams to Display.vi"("ACQUIPARAMS"=w113) -> ("ACQUIPARAMS Display"=w114:T7)
        n50 = local write "ACQUIPARAMS Display"(w114) -> ()
        n51 = local write "Parameters"(w113) -> ()
        n52 = Wait (ms)(milliseconds to wait=u32 250) -> ()  [unwired: 1 out]
      }
      frame "Capture" {
        # "Starts the Cine recording"
        n53 = property on="active" class="Str"(error in=w135, "Value"=w134) -> (error out=w133:errorcluster)  [unwired: 1 in, 1 out]
        n54 = call "Vision Research Phantom Series PhCon PhRecordCine.vi"("CN in"=w131, "Error In (no error)"=w133) -> ("Error Out"=w137:errorcluster)  [unwired: 17 out]
        n55 = Wait (ms)(milliseconds to wait=u32 250) -> ()  [unwired: 1 out]
      }
      frame "Trigger" {
        w139 = FALSE
        # "Waits post trigger frames"
        # "Sends a trigger to the cine"
        n56 = property on="active" class="Str"(error in=w150, "Value"=w148) -> (error out=w149:errorcluster)  [unwired: 1 in, 1 out]
        n57 = call "Vision Research Phantom Series PhCon PhSendTrigger.vi"("CN in"=w140, "Error In (no error)"=w149) -> ("Error Out"=w143:errorcluster)  [unwired: 17 out]
        n58 = Unbundle By Name(w145) -> ("PTFrames"=w146:u32, "(deprecated)FrameRateInt"=w147:u32)
        n59 = Divide(x=w146, y=w147) -> (x/y=w144:dbl)
        n60 = Increment(x=w144) -> (x+1=w141:dbl)
        n61 = call "Time Delay"("error in (no error)"=w143, "Delay Time (s)"=w141) -> ("error out"=w142:errorcluster)  [unwired: 9 out]
        n62 = local write "Capture"(w139) -> ()
        n63 = local write "Trigger"(w139) -> ()
      }
      frame "Open Cine" {
        n64 = case shown="1" w155 {
          tunnel: w159 -> [w233 w239]
          tunnel: [w227 w238] -> w158
          tunnel: [w226 w237] -> w157
          tunnel: w154 -> [w232 _]
          tunnel: w153 -> [w229 _]
          tunnel: [TRUE w234] -> w152
          frame 0, Default {
            n65 = call "Vision Research Phantom Series PhCon PhPhGetCineCount.vi"("CN in"=w232, "Error In (no error)"=w233) -> ("CN out"=w230:u32, "pRAMCount"=w228:u32, "Error Out"=w231:errorcluster)  [unwired: 15 out]
            n66 = property on="Cine Number" class="DigNum (strict)"("Maximum"=w228) -> ()  [unwired: 2 in, 2 out]
            n67 = call "Vision Research Phantom Series PhFile PhNewCineFromCamera.vi"("Camera Number in"=w230, "CineNr in"=w229, "Error In (no error)"=w231) -> ("pCH"=w227:u32, "Error Out"=w226:errorcluster)  [unwired: 15 out]
          }
          frame 1 {
            w240 = u32 0 items=["0", "OFN_MULTISELECT"] ("Options")
            n68 = call "Vision Research Phantom Series PhFile PhGetOpenCineName.vi"("Options"=w240, "Error In (no error)"=w239) -> ("szFileName"=w235:path, "Success"=w234:bool, "Error Out"=w236:errorcluster)  [unwired: 15 out]
            n69 = call "Vision Research Phantom Series PhFile PhNewCineFromFile.vi"("szFileName"=w235, "Error In (no error)"=w236) -> ("pCH"=w238:u32, "Error Out"=w237:errorcluster)  [unwired: 16 out]
          }
        }
        n70 = case shown="True" w152 {
          tunnel: w158 -> [_ w166]
          tunnel: w157 -> [w162 w165]
          tunnel: [w162 w163] -> w156
          frame False {
          }
          frame True {
            w172 = T14 28 items=["GCI_CFA"=0, "GCI_FRAMERATE"=1, "GCI_EXPOSURE"=2, "GCI_AUTOEXPOSURE"=3, "GCI_REALBPP"=4, "GCI_CAMERASERIAL"=5, "GCI_HEADSERIAL0"=6, "GCI_HEADSERIAL1"=7, "GCI_HEADSERIAL2"=8, "GCI_HEADSERIAL3"=9, "GCI_TRIGTIMESEC"=10, "GCI_TRIGTIMEFR"=11, "GCI_ISFILECINE"=12, "GCI_IS16BPPCINE"=13, "GCI_ISCOLORCINE"=14, "GCI_ISMULTIHEADCINE"=15, "GCI_EXPOSURENS"=16, "GCI_EDREXPOSURENS"=17, "GCI_FRAMEDELAYNS"=19, "GCI_FROMFILETYPE"=20, "GCI_COMPRESSION"=21, "GCI_CAMERAVERSION"=22, "GCI_ROTATE"=23, "GCI_IMWIDTH"=24, "GCI_IMHEIGHT"=25, "GCI_IMWIDTHACQ"=26, "GCI_IMHEIGHTACQ"=27, "GCI_POSTTRIGGER"=28, "GCI_IMAGECOUNT"=29, "GCI_TOTALIMAGECOUNT"=30, "GCI_TRIGFRAME"=31, "GCI_AUTOEXPLEVEL"=32, "GCI_AUTOEXPTOP"=33, "GCI_AUTOEXPLEFT"=34, "GCI_AUTOEXPBOTTOM"=35, "GCI_AUTOEXPRIGHT"=36, "GCI_RECORDINGTIMEZONE"=37, "GCI_FIRSTIMAGENO"=38, "GCI_FIRSTMOVIEIMAGE"=39, "GCI_CINENAME"=40, "GCI_FRPSTEPS"=100, "GCI_FRP1X"=101, "GCI_FRP1Y"=102, "GCI_FRP2X"=103, "GCI_FRP2Y"=104, "GCI_FRP3X"=105, "GCI_FRP3Y"=106, "GCI_FRP4X"=107, "GCI_FRP4Y"=108, "GCI_WRITEERR"=109, "GCI_LENSDESCRIPTION"=110, "GCI_LENSAPERATURE"=111, "GCI_LENSFOCALLENGTH"=112, "GCI_WB"=200, "GCI_WBVIEW"=201, "GCI_BRIGHT"=202, "GCI_CONTRAST"=203, "GCI_GAMMA"=204, "GCI_GAMMAR"=223, "GCI_GAMMAB"=224, "GCI_SATURATION"=205, "GCI_HUE"=206, "GCI_FLIPH"=207, "GCI_FLIPV"=208, "GCI_FILTERCODE"=209, "GCI_IMFILTER"=210, "GCI_INTALGO"=211, "GCI_PEDESTALR"=212, "GCI_PEDESTALG"=213, "GCI_PEDESTALB"=214, "GCI_FLARE"=225, "GCI_CHROMA"=226, "GCI_TONE"=227, "GCI_ENABLEMATRICES"=228, "GCI_USERMATRIX"=229, "GCI_RESAMPLEACTIVE"=215, "GCI_RESAMPLEWIDTH"=216, "GCI_RESAMPLEHEIGHT"=217, "GCI_CROPACTIVE"=218, "GCI_CROPRECTANGLE"=219, "GCI_OFFSET16_8"=220, "GCI_GAIN16_8"=221, "GCI_DEMOSAICINGFUNCPTR"=222, "GCI_VFLIPVIEWACTIVE"=300, "GCI_MAXIMGSIZE"=400, "GCI_FRPIMGNOARRAY"=450, "GCI_FRPRATEARRAY"=451, "GCI_FRPSHAPEARRAY"=452, "GCI_TRIGTC"=470, "GCI_TRIGTCU"=471, "GCI_PBRATE"=472, "GCI_TCRATE"=473, "GCI_SAVERANGE"=500, "GCI_SAVEFILENAME"=501, "GCI_SAVEFILETYPE"=502, "GCI_SAVE16BIT"=503, "GCI_SAVEPACKED"=504, "GCI_SAVEXML"=505, "GCI_SAVESTAMPTIME"=506, "GCI_SAVEAVIFRAMERATE"=520, "GCI_SAVEAVICOMPRESSORLIST"=521, "GCI_SAVEAVICOMPRESSORINDEX"=522, "GCI_SAVEDPXLSB"=530, "GCI_SAVEDPXTO10BPS"=531, "GCI_SAVEDPXDATAPACKING"=532, "GCI_SAVEDPX10BITLOG"=533, "GCI_SAVEDPXEXPORTLOGLUT"=534, "GCI_SAVEDPX10BITLOGREFWHITE"=535, "GCI_SAVEDPX10BITLOGREFBLACK"=536, "GCI_SAVEDPX10BITLOGGAMMA"=537, "GCI_SAVEDPX10BITLOGFILMGAMMA"=538, "GCI_SAVEQTPLAYBACKRATE"=550, "GCI_SAVECCIQUALITY"=560, "GCI_UNCALIBRATEDIMAGE"=600, "GCI_NOPROCESSING"=601, "GCI_BADPIXELREPAIR"=602] ("InfName")
            w173 = T14 29 items=["GCI_CFA"=0, "GCI_FRAMERATE"=1, "GCI_EXPOSURE"=2, "GCI_AUTOEXPOSURE"=3, "GCI_REALBPP"=4, "GCI_CAMERASERIAL"=5, "GCI_HEADSERIAL0"=6, "GCI_HEADSERIAL1"=7, "GCI_HEADSERIAL2"=8, "GCI_HEADSERIAL3"=9, "GCI_TRIGTIMESEC"=10, "GCI_TRIGTIMEFR"=11, "GCI_ISFILECINE"=12, "GCI_IS16BPPCINE"=13, "GCI_ISCOLORCINE"=14, "GCI_ISMULTIHEADCINE"=15, "GCI_EXPOSURENS"=16, "GCI_EDREXPOSURENS"=17, "GCI_FRAMEDELAYNS"=19, "GCI_FROMFILETYPE"=20, "GCI_COMPRESSION"=21, "GCI_CAMERAVERSION"=22, "GCI_ROTATE"=23, "GCI_IMWIDTH"=24, "GCI_IMHEIGHT"=25, "GCI_IMWIDTHACQ"=26, "GCI_IMHEIGHTACQ"=27, "GCI_POSTTRIGGER"=28, "GCI_IMAGECOUNT"=29, "GCI_TOTALIMAGECOUNT"=30, "GCI_TRIGFRAME"=31, "GCI_AUTOEXPLEVEL"=32, "GCI_AUTOEXPTOP"=33, "GCI_AUTOEXPLEFT"=34, "GCI_AUTOEXPBOTTOM"=35, "GCI_AUTOEXPRIGHT"=36, "GCI_RECORDINGTIMEZONE"=37, "GCI_FIRSTIMAGENO"=38, "GCI_FIRSTMOVIEIMAGE"=39, "GCI_CINENAME"=40, "GCI_FRPSTEPS"=100, "GCI_FRP1X"=101, "GCI_FRP1Y"=102, "GCI_FRP2X"=103, "GCI_FRP2Y"=104, "GCI_FRP3X"=105, "GCI_FRP3Y"=106, "GCI_FRP4X"=107, "GCI_FRP4Y"=108, "GCI_WRITEERR"=109, "GCI_LENSDESCRIPTION"=110, "GCI_LENSAPERATURE"=111, "GCI_LENSFOCALLENGTH"=112, "GCI_WB"=200, "GCI_WBVIEW"=201, "GCI_BRIGHT"=202, "GCI_CONTRAST"=203, "GCI_GAMMA"=204, "GCI_GAMMAR"=223, "GCI_GAMMAB"=224, "GCI_SATURATION"=205, "GCI_HUE"=206, "GCI_FLIPH"=207, "GCI_FLIPV"=208, "GCI_FILTERCODE"=209, "GCI_IMFILTER"=210, "GCI_INTALGO"=211, "GCI_PEDESTALR"=212, "GCI_PEDESTALG"=213, "GCI_PEDESTALB"=214, "GCI_FLARE"=225, "GCI_CHROMA"=226, "GCI_TONE"=227, "GCI_ENABLEMATRICES"=228, "GCI_USERMATRIX"=229, "GCI_RESAMPLEACTIVE"=215, "GCI_RESAMPLEWIDTH"=216, "GCI_RESAMPLEHEIGHT"=217, "GCI_CROPACTIVE"=218, "GCI_CROPRECTANGLE"=219, "GCI_OFFSET16_8"=220, "GCI_GAIN16_8"=221, "GCI_DEMOSAICINGFUNCPTR"=222, "GCI_VFLIPVIEWACTIVE"=300, "GCI_MAXIMGSIZE"=400, "GCI_FRPIMGNOARRAY"=450, "GCI_FRPRATEARRAY"=451, "GCI_FRPSHAPEARRAY"=452, "GCI_TRIGTC"=470, "GCI_TRIGTCU"=471, "GCI_PBRATE"=472, "GCI_TCRATE"=473, "GCI_SAVERANGE"=500, "GCI_SAVEFILENAME"=501, "GCI_SAVEFILETYPE"=502, "GCI_SAVE16BIT"=503, "GCI_SAVEPACKED"=504, "GCI_SAVEXML"=505, "GCI_SAVESTAMPTIME"=506, "GCI_SAVEAVIFRAMERATE"=520, "GCI_SAVEAVICOMPRESSORLIST"=521, "GCI_SAVEAVICOMPRESSORINDEX"=522, "GCI_SAVEDPXLSB"=530, "GCI_SAVEDPXTO10BPS"=531, "GCI_SAVEDPXDATAPACKING"=532, "GCI_SAVEDPX10BITLOG"=533, "GCI_SAVEDPXEXPORTLOGLUT"=534, "GCI_SAVEDPX10BITLOGREFWHITE"=535, "GCI_SAVEDPX10BITLOGREFBLACK"=536, "GCI_SAVEDPX10BITLOGGAMMA"=537, "GCI_SAVEDPX10BITLOGFILMGAMMA"=538, "GCI_SAVEQTPLAYBACKRATE"=550, "GCI_SAVECCIQUALITY"=560, "GCI_UNCALIBRATEDIMAGE"=600, "GCI_NOPROCESSING"=601, "GCI_BADPIXELREPAIR"=602] ("InfName")
            n71 = call "Vision Research Phantom Series PhFile PhGetCineInfo.vi"("CH in"=w166, "InfName"=w173, "Error In (no error)"=w165) -> ("CH out"=w170:u32, "pInfVal out"=w164:i32, "Error Out"=w171:errorcluster)  [unwired: 14 out]
            "Image Count" <- w164
            n72 = call "Vision Research Phantom Series PhFile PhGetCineInfo.vi"("CH in"=w170, "InfName"=w172, "Error In (no error)"=w171) -> ("CH out"=w169:u32, "pInfVal out"=w167:i32, "Error Out"=w168:errorcluster)  [unwired: 14 out]
            "Post-Trigger Frames" <- w167
            n73 = while {
              tunnel: w168 -> [w182]
              tunnel: w167 -> [w180]
              tunnel: w164 -> [w176]
              tunnel: [w179] -> w163
              tunnel: w164 -> [w175]
              tunnel: w169 -> [w177]
              stop <- w178 stop-if-true
              n74 = Subtract(x=w180, y=w175) -> (x-y=w181:i32)
              n75 = for {
                N: w176 -> [_]
                tunnel: w182 -> [w203]
                tunnel: w181 -> [w192]
                tunnel: [w208] -> w179
                tunnel: [w190] -> w178
                tunnel: w177 -> [w184]
                tunnel: "Delay (ms)" -> [w193]
                i -> [w213]
                stop <- w190 stop-if-true
                w189 = T14 14 items=["GCI_CFA"=0, "GCI_FRAMERATE"=1, "GCI_EXPOSURE"=2, "GCI_AUTOEXPOSURE"=3, "GCI_REALBPP"=4, "GCI_CAMERASERIAL"=5, "GCI_HEADSERIAL0"=6, "GCI_HEADSERIAL1"=7, "GCI_HEADSERIAL2"=8, "GCI_HEADSERIAL3"=9, "GCI_TRIGTIMESEC"=10, "GCI_TRIGTIMEFR"=11, "GCI_ISFILECINE"=12, "GCI_IS16BPPCINE"=13, "GCI_ISCOLORCINE"=14, "GCI_ISMULTIHEADCINE"=15, "GCI_EXPOSURENS"=16, "GCI_EDREXPOSURENS"=17, "GCI_FRAMEDELAYNS"=19, "GCI_FROMFILETYPE"=20, "GCI_COMPRESSION"=21, "GCI_CAMERAVERSION"=22, "GCI_ROTATE"=23, "GCI_IMWIDTH"=24, "GCI_IMHEIGHT"=25, "GCI_IMWIDTHACQ"=26, "GCI_IMHEIGHTACQ"=27, "GCI_POSTTRIGGER"=28, "GCI_IMAGECOUNT"=29, "GCI_TOTALIMAGECOUNT"=30, "GCI_TRIGFRAME"=31, "GCI_AUTOEXPLEVEL"=32, "GCI_AUTOEXPTOP"=33, "GCI_AUTOEXPLEFT"=34, "GCI_AUTOEXPBOTTOM"=35, "GCI_AUTOEXPRIGHT"=36, "GCI_RECORDINGTIMEZONE"=37, "GCI_FIRSTIMAGENO"=38, "GCI_FIRSTMOVIEIMAGE"=39, "GCI_CINENAME"=40, "GCI_FRPSTEPS"=100, "GCI_FRP1X"=101, "GCI_FRP1Y"=102, "GCI_FRP2X"=103, "GCI_FRP2Y"=104, "GCI_FRP3X"=105, "GCI_FRP3Y"=106, "GCI_FRP4X"=107, "GCI_FRP4Y"=108, "GCI_WRITEERR"=109, "GCI_LENSDESCRIPTION"=110, "GCI_LENSAPERATURE"=111, "GCI_LENSFOCALLENGTH"=112, "GCI_WB"=200, "GCI_WBVIEW"=201, "GCI_BRIGHT"=202, "GCI_CONTRAST"=203, "GCI_GAMMA"=204, "GCI_GAMMAR"=223, "GCI_GAMMAB"=224, "GCI_SATURATION"=205, "GCI_HUE"=206, "GCI_FLIPH"=207, "GCI_FLIPV"=208, "GCI_FILTERCODE"=209, "GCI_IMFILTER"=210, "GCI_INTALGO"=211, "GCI_PEDESTALR"=212, "GCI_PEDESTALG"=213, "GCI_PEDESTALB"=214, "GCI_FLARE"=225, "GCI_CHROMA"=226, "GCI_TONE"=227, "GCI_ENABLEMATRICES"=228, "GCI_USERMATRIX"=229, "GCI_RESAMPLEACTIVE"=215, "GCI_RESAMPLEWIDTH"=216, "GCI_RESAMPLEHEIGHT"=217, "GCI_CROPACTIVE"=218, "GCI_CROPRECTANGLE"=219, "GCI_OFFSET16_8"=220, "GCI_GAIN16_8"=221, "GCI_DEMOSAICINGFUNCPTR"=222, "GCI_VFLIPVIEWACTIVE"=300, "GCI_MAXIMGSIZE"=400, "GCI_FRPIMGNOARRAY"=450, "GCI_FRPRATEARRAY"=451, "GCI_FRPSHAPEARRAY"=452, "GCI_TRIGTC"=470, "GCI_TRIGTCU"=471, "GCI_PBRATE"=472, "GCI_TCRATE"=473, "GCI_SAVERANGE"=500, "GCI_SAVEFILENAME"=501, "GCI_SAVEFILETYPE"=502, "GCI_SAVE16BIT"=503, "GCI_SAVEPACKED"=504, "GCI_SAVEXML"=505, "GCI_SAVESTAMPTIME"=506, "GCI_SAVEAVIFRAMERATE"=520, "GCI_SAVEAVICOMPRESSORLIST"=521, "GCI_SAVEAVICOMPRESSORINDEX"=522, "GCI_SAVEDPXLSB"=530, "GCI_SAVEDPXTO10BPS"=531, "GCI_SAVEDPXDATAPACKING"=532, "GCI_SAVEDPX10BITLOG"=533, "GCI_SAVEDPXEXPORTLOGLUT"=534, "GCI_SAVEDPX10BITLOGREFWHITE"=535, "GCI_SAVEDPX10BITLOGREFBLACK"=536, "GCI_SAVEDPX10BITLOGGAMMA"=537, "GCI_SAVEDPX10BITLOGFILMGAMMA"=538, "GCI_SAVEQTPLAYBACKRATE"=550, "GCI_SAVECCIQUALITY"=560, "GCI_UNCALIBRATEDIMAGE"=600, "GCI_NOPROCESSING"=601, "GCI_BADPIXELREPAIR"=602] ("InfName")
                w200 = T14 400 items=["GCI_CFA"=0, "GCI_FRAMERATE"=1, "GCI_EXPOSURE"=2, "GCI_AUTOEXPOSURE"=3, "GCI_REALBPP"=4, "GCI_CAMERASERIAL"=5, "GCI_HEADSERIAL0"=6, "GCI_HEADSERIAL1"=7, "GCI_HEADSERIAL2"=8, "GCI_HEADSERIAL3"=9, "GCI_TRIGTIMESEC"=10, "GCI_TRIGTIMEFR"=11, "GCI_ISFILECINE"=12, "GCI_IS16BPPCINE"=13, "GCI_ISCOLORCINE"=14, "GCI_ISMULTIHEADCINE"=15, "GCI_EXPOSURENS"=16, "GCI_EDREXPOSURENS"=17, "GCI_FRAMEDELAYNS"=19, "GCI_FROMFILETYPE"=20, "GCI_COMPRESSION"=21, "GCI_CAMERAVERSION"=22, "GCI_ROTATE"=23, "GCI_IMWIDTH"=24, "GCI_IMHEIGHT"=25, "GCI_IMWIDTHACQ"=26, "GCI_IMHEIGHTACQ"=27, "GCI_POSTTRIGGER"=28, "GCI_IMAGECOUNT"=29, "GCI_TOTALIMAGECOUNT"=30, "GCI_TRIGFRAME"=31, "GCI_AUTOEXPLEVEL"=32, "GCI_AUTOEXPTOP"=33, "GCI_AUTOEXPLEFT"=34, "GCI_AUTOEXPBOTTOM"=35, "GCI_AUTOEXPRIGHT"=36, "GCI_RECORDINGTIMEZONE"=37, "GCI_FIRSTIMAGENO"=38, "GCI_FIRSTMOVIEIMAGE"=39, "GCI_CINENAME"=40, "GCI_FRPSTEPS"=100, "GCI_FRP1X"=101, "GCI_FRP1Y"=102, "GCI_FRP2X"=103, "GCI_FRP2Y"=104, "GCI_FRP3X"=105, "GCI_FRP3Y"=106, "GCI_FRP4X"=107, "GCI_FRP4Y"=108, "GCI_WRITEERR"=109, "GCI_LENSDESCRIPTION"=110, "GCI_LENSAPERATURE"=111, "GCI_LENSFOCALLENGTH"=112, "GCI_WB"=200, "GCI_WBVIEW"=201, "GCI_BRIGHT"=202, "GCI_CONTRAST"=203, "GCI_GAMMA"=204, "GCI_GAMMAR"=223, "GCI_GAMMAB"=224, "GCI_SATURATION"=205, "GCI_HUE"=206, "GCI_FLIPH"=207, "GCI_FLIPV"=208, "GCI_FILTERCODE"=209, "GCI_IMFILTER"=210, "GCI_INTALGO"=211, "GCI_PEDESTALR"=212, "GCI_PEDESTALG"=213, "GCI_PEDESTALB"=214, "GCI_FLARE"=225, "GCI_CHROMA"=226, "GCI_TONE"=227, "GCI_ENABLEMATRICES"=228, "GCI_USERMATRIX"=229, "GCI_RESAMPLEACTIVE"=215, "GCI_RESAMPLEWIDTH"=216, "GCI_RESAMPLEHEIGHT"=217, "GCI_CROPACTIVE"=218, "GCI_CROPRECTANGLE"=219, "GCI_OFFSET16_8"=220, "GCI_GAIN16_8"=221, "GCI_DEMOSAICINGFUNCPTR"=222, "GCI_VFLIPVIEWACTIVE"=300, "GCI_MAXIMGSIZE"=400, "GCI_FRPIMGNOARRAY"=450, "GCI_FRPRATEARRAY"=451, "GCI_FRPSHAPEARRAY"=452, "GCI_TRIGTC"=470, "GCI_TRIGTCU"=471, "GCI_PBRATE"=472, "GCI_TCRATE"=473, "GCI_SAVERANGE"=500, "GCI_SAVEFILENAME"=501, "GCI_SAVEFILETYPE"=502, "GCI_SAVE16BIT"=503, "GCI_SAVEPACKED"=504, "GCI_SAVEXML"=505, "GCI_SAVESTAMPTIME"=506, "GCI_SAVEAVIFRAMERATE"=520, "GCI_SAVEAVICOMPRESSORLIST"=521, "GCI_SAVEAVICOMPRESSORINDEX"=522, "GCI_SAVEDPXLSB"=530, "GCI_SAVEDPXTO10BPS"=531, "GCI_SAVEDPXDATAPACKING"=532, "GCI_SAVEDPX10BITLOG"=533, "GCI_SAVEDPXEXPORTLOGLUT"=534, "GCI_SAVEDPX10BITLOGREFWHITE"=535, "GCI_SAVEDPX10BITLOGREFBLACK"=536, "GCI_SAVEDPX10BITLOGGAMMA"=537, "GCI_SAVEDPX10BITLOGFILMGAMMA"=538, "GCI_SAVEQTPLAYBACKRATE"=550, "GCI_SAVECCIQUALITY"=560, "GCI_UNCALIBRATEDIMAGE"=600, "GCI_NOPROCESSING"=601, "GCI_BADPIXELREPAIR"=602] ("InfName")
                w207 = T13 1 items=["IMG_PROC_REDUCE16TO8"=1] ("procID")
                n76 = call "Vision Research Phantom Series PhFile PhGetCineInfo.vi"("CH in"=w184, "InfName"=w200, "Error In (no error)"=w203) -> ("CH out"=w201:u32, "pInfVal out"=w199:i32, "Error Out"=w202:errorcluster)  [unwired: 14 out]
                n77 = Wait (ms)(milliseconds to wait=w193) -> ()  [unwired: 1 out]
                n78 = Add(x=w192, y=w213) -> (x+y=w196:i32)
                "Current Image #" <- w196
                n79 = Initialize Array(u16 0 ("element"), w199) -> (w210:u16[])
                n80 = Bundle By Name(cluster=T11 {"First"=0, "Cnt"=1} ("pRng"), "First"=w196) -> (w211:T11)
                n81 = call "Vision Research Phantom Series PhFile PhGetCineImage.vi"("hC [in]"=w201, "pRng [in]"=w211, "bufferByteSize [in]"=w199, "pPixelBuffer [in]"=w210, "Error In (no error)"=w202) -> ("pPixelBuffer [out]"=w206:u16[], "IH [out]"=w205:T15, "Error Out"=w204:errorcluster)  [unwired: 12 out]
                n82 = while {
                  tunnel: ["Preview Img"] -> w190
                  stop <- w222 continue-if-true
                  n83 = Not(x="Preview Img") -> (.not. x?=w223:bool)
                  n84 = And(x=w223, y="Play/Pause") -> (x .and. y?=w222:bool)
                }
                n85 = Absolute Value(x=w192) -> (abs(x)=w191:i32)
                n86 = call "Vision Research Phantom Series PhInt PhProcessImage.vi"("pPixelSrc [in]"=w206, "IH [in]"=w205, "procID"=w207, "pProcParams"=1.0, "Error In (no error)"=w204) -> ("pPixelDest [out]"=w186:u8[], "IH [out]"=w183:T15, "Error Out"=w185:errorcluster)  [unwired: 12 out]
                n87 = call "Vision Research Phantom Series PhFile PhGetCineInfo.vi"("CH in"=w184, "InfName"=w189, "Error In (no error)"=w185) -> ("pInfVal out"=w188:i32)  [unwired: 16 out]
                n88 = case shown="1, Default" w188 {
                  tunnel: [w215 w217] -> w187
                  tunnel: w186 -> [w215 w216]
                  frame 0 {
                  }
                  frame 1, Default {
                    n89 = Decimate 1D Array(w216) -> (w220:u8[], w219:u8[], w218:u8[])
                    n90 = Interleave 1D Arrays(w218, w219, w220) -> (w217:u8[])
                  }
                }
                n91 = Add(x=w191, y=w196) -> (x+y=w195:i32)
                n92 = Divide(x=w195, y=w191) -> (x/y=→"Slide":dbl)
                n93 = call "Vision Research Phantom Series PhInt PhIHtoBITMAPINFOHEADER.vi"("IH"=w183) -> ("BITMAPINFOHEADER"=w209:T16, "Error Out"=w208:errorcluster)  [unwired: 1 in, 16 out]
                n94 = call "pPixel to Picture.vi"("pPixel"=w187, "BITMAPINFOHEADER"=w209) -> ("Preview"=w198:picture)  [unwired: 1 in]
                n95 = local write "Preview"(w198) -> ()
              }
            }
          }
        }
      }
      frame "Save Cine" {
        w254 = T14 506 items=["GCI_CFA"=0, "GCI_FRAMERATE"=1, "GCI_EXPOSURE"=2, "GCI_AUTOEXPOSURE"=3, "GCI_REALBPP"=4, "GCI_CAMERASERIAL"=5, "GCI_HEADSERIAL0"=6, "GCI_HEADSERIAL1"=7, "GCI_HEADSERIAL2"=8, "GCI_HEADSERIAL3"=9, "GCI_TRIGTIMESEC"=10, "GCI_TRIGTIMEFR"=11, "GCI_ISFILECINE"=12, "GCI_IS16BPPCINE"=13, "GCI_ISCOLORCINE"=14, "GCI_ISMULTIHEADCINE"=15, "GCI_EXPOSURENS"=16, "GCI_EDREXPOSURENS"=17, "GCI_FRAMEDELAYNS"=19, "GCI_FROMFILETYPE"=20, "GCI_COMPRESSION"=21, "GCI_CAMERAVERSION"=22, "GCI_ROTATE"=23, "GCI_IMWIDTH"=24, "GCI_IMHEIGHT"=25, "GCI_IMWIDTHACQ"=26, "GCI_IMHEIGHTACQ"=27, "GCI_POSTTRIGGER"=28, "GCI_IMAGECOUNT"=29, "GCI_TOTALIMAGECOUNT"=30, "GCI_TRIGFRAME"=31, "GCI_AUTOEXPLEVEL"=32, "GCI_AUTOEXPTOP"=33, "GCI_AUTOEXPLEFT"=34, "GCI_AUTOEXPBOTTOM"=35, "GCI_AUTOEXPRIGHT"=36, "GCI_RECORDINGTIMEZONE"=37, "GCI_FIRSTIMAGENO"=38, "GCI_FIRSTMOVIEIMAGE"=39, "GCI_CINENAME"=40, "GCI_FRPSTEPS"=100, "GCI_FRP1X"=101, "GCI_FRP1Y"=102, "GCI_FRP2X"=103, "GCI_FRP2Y"=104, "GCI_FRP3X"=105, "GCI_FRP3Y"=106, "GCI_FRP4X"=107, "GCI_FRP4Y"=108, "GCI_WRITEERR"=109, "GCI_LENSDESCRIPTION"=110, "GCI_LENSAPERATURE"=111, "GCI_LENSFOCALLENGTH"=112, "GCI_WB"=200, "GCI_WBVIEW"=201, "GCI_BRIGHT"=202, "GCI_CONTRAST"=203, "GCI_GAMMA"=204, "GCI_GAMMAR"=223, "GCI_GAMMAB"=224, "GCI_SATURATION"=205, "GCI_HUE"=206, "GCI_FLIPH"=207, "GCI_FLIPV"=208, "GCI_FILTERCODE"=209, "GCI_IMFILTER"=210, "GCI_INTALGO"=211, "GCI_PEDESTALR"=212, "GCI_PEDESTALG"=213, "GCI_PEDESTALB"=214, "GCI_FLARE"=225, "GCI_CHROMA"=226, "GCI_TONE"=227, "GCI_ENABLEMATRICES"=228, "GCI_USERMATRIX"=229, "GCI_RESAMPLEACTIVE"=215, "GCI_RESAMPLEWIDTH"=216, "GCI_RESAMPLEHEIGHT"=217, "GCI_CROPACTIVE"=218, "GCI_CROPRECTANGLE"=219, "GCI_OFFSET16_8"=220, "GCI_GAIN16_8"=221, "GCI_DEMOSAICINGFUNCPTR"=222, "GCI_VFLIPVIEWACTIVE"=300, "GCI_MAXIMGSIZE"=400, "GCI_FRPIMGNOARRAY"=450, "GCI_FRPRATEARRAY"=451, "GCI_FRPSHAPEARRAY"=452, "GCI_TRIGTC"=470, "GCI_TRIGTCU"=471, "GCI_PBRATE"=472, "GCI_TCRATE"=473, "GCI_SAVERANGE"=500, "GCI_SAVEFILENAME"=501, "GCI_SAVEFILETYPE"=502, "GCI_SAVE16BIT"=503, "GCI_SAVEPACKED"=504, "GCI_SAVEXML"=505, "GCI_SAVESTAMPTIME"=506, "GCI_SAVEAVIFRAMERATE"=520, "GCI_SAVEAVICOMPRESSORLIST"=521, "GCI_SAVEAVICOMPRESSORINDEX"=522, "GCI_SAVEDPXLSB"=530, "GCI_SAVEDPXTO10BPS"=531, "GCI_SAVEDPXDATAPACKING"=532, "GCI_SAVEDPX10BITLOG"=533, "GCI_SAVEDPXEXPORTLOGLUT"=534, "GCI_SAVEDPX10BITLOGREFWHITE"=535, "GCI_SAVEDPX10BITLOGREFBLACK"=536, "GCI_SAVEDPX10BITLOGGAMMA"=537, "GCI_SAVEDPX10BITLOGFILMGAMMA"=538, "GCI_SAVEQTPLAYBACKRATE"=550, "GCI_SAVECCIQUALITY"=560, "GCI_UNCALIBRATEDIMAGE"=600, "GCI_NOPROCESSING"=601, "GCI_BADPIXELREPAIR"=602] ("InfName [in]")
        w241 = FALSE
        # "Saves Cine to file"
        n96 = property on="active" class="Str"(error in=w256, "Value"=w255) -> (error out=w248:errorcluster)  [unwired: 1 in, 1 out]
        n97 = call "Vision Research Phantom Series PhFile PhNewCineFromCamera.vi"("Camera Number in"=w247, "CineNr in"=1, "Error In (no error)"=w248) -> ("pCH"=w244:u32, "Error Out"=w243:errorcluster)  [unwired: 1 in, 14 out]
        n98 = call "Vision Research Phantom Series PhFile PhSetCineInfo.vi"("CH [in]"=w244, "InfName [in]"=w254, "pInfVal [in]"="Save StampTime", "Error In (no error)"=w243) -> ("CH [out]"=w251:u32, "Error Out"=w252:errorcluster)  [unwired: 14 out]
        n99 = call "Vision Research Phantom Series PhFile PhGetSaveCineName.vi"("CH in"=w251, "Error In (no error)"=w252) -> ("CH out"=w249:u32, "Success"=w242:bool, "Error Out"=w250:errorcluster)  [unwired: 15 out]
        n100 = case shown="True" w242 {
          tunnel: w250 -> [w258 w261]
          tunnel: w249 -> [_ w260]
          tunnel: [w258 w259] -> w245
          frame False {
          }
          frame True {
            n101 = while {
              tunnel: w261 -> [w267]
              tunnel: w260 -> [w266]
              stop <- w264 continue-if-true
              n102 = call "Vision Research Phantom Series PhFile PhGetWriteCineFileProgress.vi"("CH [in]"=w266, "Error In (no error)"=w267) -> ("pProgressPercent [out]"=w263:u32, "Error Out"=w265:errorcluster)  [unwired: 16 out]
              n103 = Wait (ms)(milliseconds to wait=u32 100) -> ()  [unwired: 1 out]
              n104 = local write "Save Progress"(w263) -> ()
              n105 = case shown="No Error" w265 {
                tunnel: [TRUE FALSE] -> w264
                frame No Error {
                }
                frame Error {
                }
              }
            }
            n106 = call "Vision Research Phantom Series PhFile PhWriteCineFile.vi"("CH in"=w260, "Error In (no error)"=w261) -> ("Error Out"=w259:errorcluster)  [unwired: 1 in, 16 out]
          }
        }
        n107 = local write "Save Cine"(w241) -> ()
      }
      frame "End" {
        w273 = FALSE ("Continue")
        # "Exits program"
        n108 = local write "Preview Img"(FALSE ("Preview Img")) -> ()
        n109 = call "Vision Research Phantom Series Close.vi"("Error In (no error)"=w275) -> ("Error Out"=w274:errorcluster)  [unwired: 18 out]
        n110 = local write "EXIT"(w273) -> ()
        n111 = local write "Image Count"(u32 0 ("Image Count")) -> ()
        n112 = local write "Play/Pause"(FALSE ("Play/Pause")) -> ()
        "Continue" <- w273
      }
    }
  }
  "error out" <- w2
